vi "Density Sensor Range--constant.vi"() -> (2 "Sensor Min":dbl, 3 "Sensor Max":dbl)   [LabVIEW 2024, in "Hardware Controller.lvlib"]
uses:
  Hardware Controller.lvlib
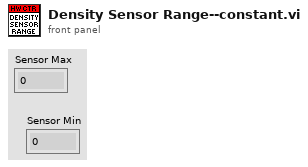
[diagram p1: front panel]
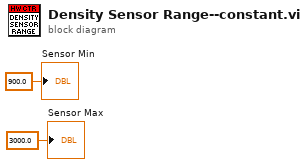
[diagram p0: block diagram]
diagram:
  "Sensor Min" <- 900.0 ("Sensor Min")
  "Sensor Max" <- 3000.0 ("Sensor Max")
